vi "WritingAttributes.vi"(0 "reference in":refnum<class "MyG#G3SubTempl.lvclass">, 1 "increment":dbl, 5 "error in (no error)":errorcluster) -> (14 "reference out":refnum<class "MyG#G3SubTempl.lvclass">, 19 "error out":errorcluster)   [LabVIEW 2020, in "MyG#G3SubTempl.lvclass"]
uses:
  MyG#G3SubTempl.lvclass
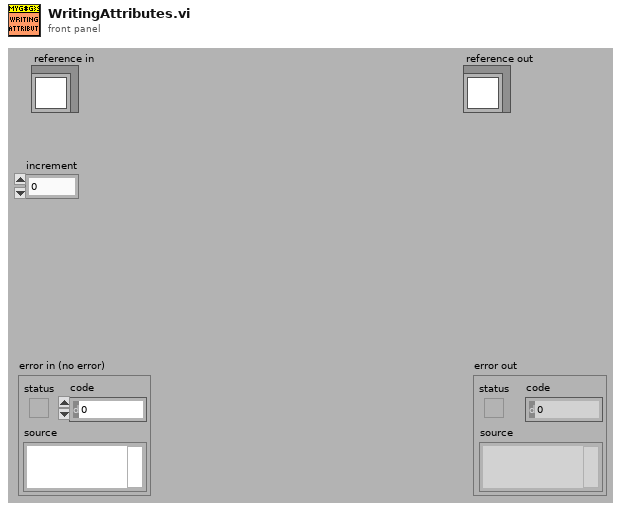
[diagram p1: front panel]
types:
  T1 = typedef "MyG#G3SubTempl.lvclass/ObjectAttributes.ctl" = cluster{"Base class":T2, "MySubAttribute":dbl}
  T2 = typedef "MyG#G3Templ.lvclass/ObjectAttributes.ctl" = cluster{"MyAttribute":dbl}
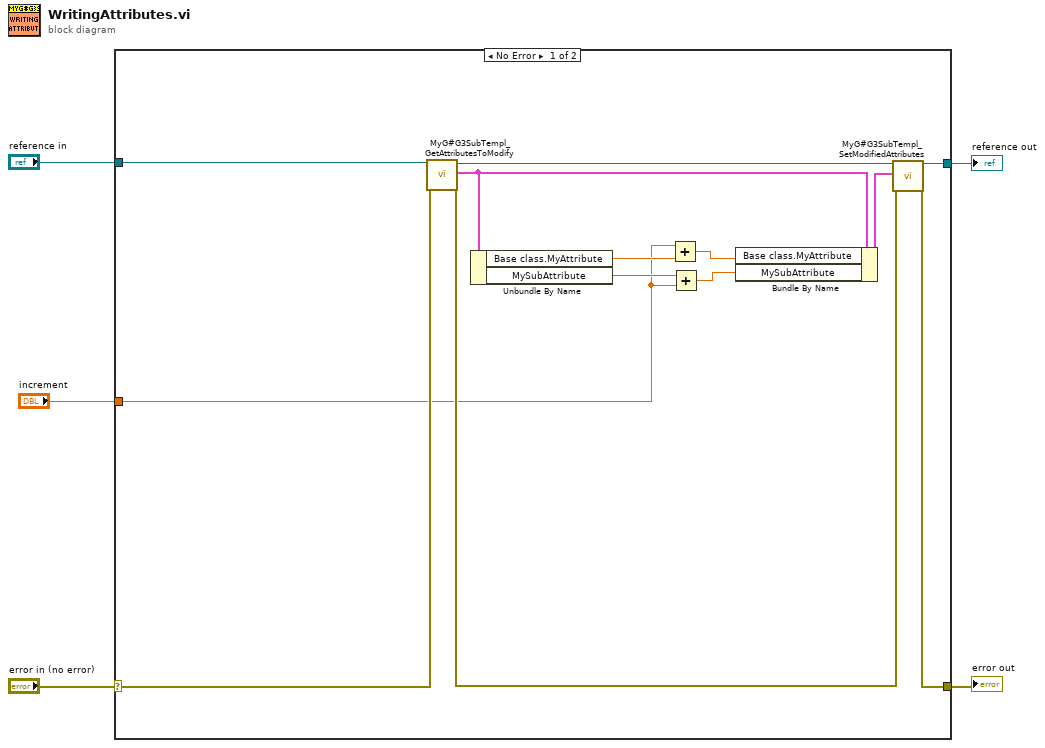
[diagram p0: block diagram]
diagram:
  n1 = case shown="No Error" "error in (no error)" {
    selector: "error in (no error)" -> [w14 w20]
    tunnel: [w16 w20] -> w4
    tunnel: [w13 w19] -> w2
    tunnel: "reference in" -> [w15 w19]
    tunnel: "increment" -> [w6 _]
    frame No Error {
      n2 = call "MyG#G3SubTempl_GetAttributesToModify.vi"("reference in"=w15, "error in (no error)"=w14) -> ("reference out"=w17:refnum<class "MyG#G3SubTempl.lvclass">, "attributes"=w11:T1, "error out"=w12:errorcluster)  [unwired: 13 in, 2 out]
      n3 = Unbundle By Name(w11) -> ("Base class.MyAttribute"=w10:dbl, "MySubAttribute"=w8:dbl)
      n4 = Add(x=w6, y=w10) -> (x+y=w9:dbl)
      n5 = Add(x=w8, y=w6) -> (x+y=w7:dbl)
      n6 = Bundle By Name(cluster=w11, "Base class.MyAttribute"=w9, "MySubAttribute"=w7) -> (w18:T1)
      n7 = call "MyG#G3SubTempl_SetModifiedAttributes.vi"("reference in"=w17, "attributes"=w18, "error in (no error)"=w12) -> ("reference out"=w13:refnum<class "MyG#G3SubTempl.lvclass">, "error out"=w16:errorcluster)  [unwired: 15 in]
    }
    frame Error {
    }
  }
  "error out" <- w4
  "reference out" <- w2
